vi "GetImagetoIMAQ.vi"(8 "error in (no error)":errorcluster, 10 "Image Src":T1, 11 "Image Data":T2) -> (0 "error out":errorcluster, 3 "Image Out":T1)   [LabVIEW 2014]
uses:
  <vilib>/picture/picture.llb/imagedata.ctl
  <vilib>/vision/Image Controls.llb/IMAQ Image.ctl
  <vilib>/vision/NI_Vision_Development_Module.lvlib
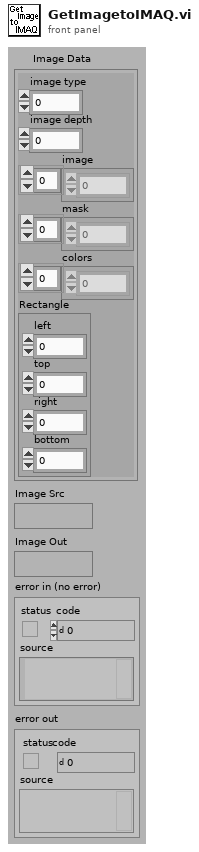
[diagram p1: front panel]
types:
  T1 = typedef "IMAQ Image.ctl" = refnum<image>
  T2 = typedef "imagedata.ctl" = cluster{"image type":i32, "image depth":i32, "image":u8[], "mask":u8[], "colors":u32[], "Rectangle":cluster{"left":i16, "top":i16, "right":i16, "bottom":i16}}
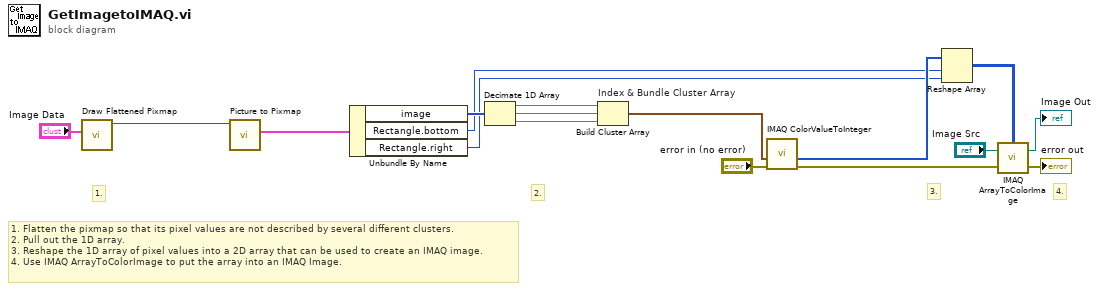
[diagram p0: block diagram]
diagram:
  # "1. Flatten the pixmap so that its pixel values are not described by several different clusters.\n2. Pull out the 1D array.\n3. Reshape the 1D array of pixel values into a 2D array that can be used to create an IMAQ image.\n4. Use IMAQ ArrayToColorImage to put the array into an IMAQ Image."
  # "4."
  # "3."
  # "2."
  # "1."
  n1 = call <vilib>:"Draw Flattened Pixmap.vi"("image data"="Image Data") -> ("new picture"=w17:picture)  [unwired: 8 in]
  n2 = call <vilib>:"Picture to Pixmap.vi"("picture"=w17) -> ("image data"=w15:T2)  [unwired: 9 in, 1 out]
  n3 = Unbundle By Name "Unbundle By Name"(w15) -> ("image"=w14:u8[], "Rectangle.bottom"=w8:i16, "Rectangle.right"=w7:i16)
  n4 = Decimate 1D Array "Decimate 1D Array"(w14) -> (w13:u8[], w12:u8[], w11:u8[])
  n5 = Build Cluster Array "Index & Bundle Cluster Array"(w13, w12, w11) -> (w10:cluster{u8, u8, u8}[])
  n6 = call "IMAQ ColorValueToInteger"("error in (no error)"="error in (no error)", "1D Color value array"=w10) -> ("1D U32 array"=w9:u32[], "error out"=w2:errorcluster)  [unwired: 3 in, 2 out]
  n7 = Reshape Array(w9, w8, w7) -> (w6:u32[][])
  n8 = call "IMAQ ArrayToColorImage"("Image Pixels (U32)"=w6, "Image"="Image Src", "error in (no error)"=w2) -> ("Image Out"=→"Image Out":T1, "error out"=→"error out":errorcluster)  [unwired: 2 in]
